vi "Read Topic Filter.vi"(8 "error in (no error)":errorcluster, 11 "Subscription in":refnum<class "Subscription.lvclass">) -> (0 "error out":errorcluster, 1 "Instance":refnum<class "TopicFilter.lvclass">, 2 "Topic Filter":string, 3 "Subscription out":refnum<class "Subscription.lvclass">)   [LabVIEW 2013, in "MQTT Base.lvlib" / "Subscription.lvclass"]
uses:
  Subscription.lvclass
  TopicFilter/TopicFilter.lvclass
  Subscription.lvclass/Subscription.ctl
  TopicFilter/TopicFilter.lvclass/TopicFilter.ctl
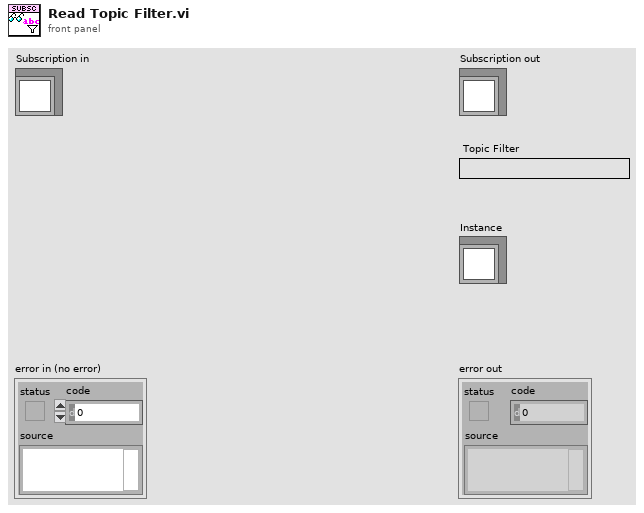
[diagram p1: front panel]
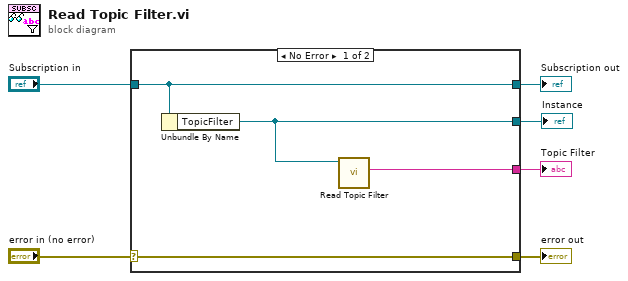
[diagram p0: block diagram]
diagram:
  n1 = case shown="No Error" "error in (no error)" {
    selector: "error in (no error)" -> [w10 w11]
    tunnel: [w10 w11] -> w5
    tunnel: [w8 w12] -> w3
    tunnel: "Subscription in" -> [w8 w12]
    tunnel: [w9 _] -> w2
    tunnel: [w7 _] -> w1
    frame No Error {
      n2 = Unbundle By Name(w8) -> ("TopicFilter"=w7:refnum<class "TopicFilter.lvclass">)
      n3 = call "Read Topic Filter.vi"("TopicFilter in"=w7) -> ("Topic Filter"=w9:string)  [unwired: 9 in, 1 out]
    }
    frame Error {
    }
  }
  "error out" <- w5
  "Subscription out" <- w3
  "Topic Filter" <- w2
  "Instance" <- w1
